vi "Pulse RFSG.vi"(0 "Test Configuration":T5, 5 "RFmx Settings":T1={"Center Frequency (Hz)"=10000000000.0, "Measurement Bandwidth (Hz)"=80000000.0, "Reference Level (dBm)"=10.0, "RFmx De-embedding"={"RFmx Name"="5842_0", "RFmx Port"="", "Attenuation"={"Mode"=enum."Constant Attenuation", "Constant Attenuation"={"RFmx External Attenuation (dB)"=1.2}, "s2p File"={"RFmx S-Parameters Orientation"=24000, "RFmx Attenuation s2p Path Name"="", "RFmx Attenuation s2p File"=path ""}}}, "Acquisition Length (s)"=0.0} {"RFmx De-embedding"."Attenuation"."s2p File"."RFmx S-Parameters Orientation" items=["Port1 Towards DUT"=24000, "Port2 Towards DUT"=24001]; "RFmx De-embedding"."Attenuation"."Constant Attenuation"."RFmx External Attenuation (dB)" format="%.2f"; "Reference Level (dBm)" format="%.2f"; "Measurement Bandwidth (Hz)" format="%.3p"; "Center Frequency (Hz)" format="%.6p"}, 7 "RFSG settings":T3={"RFSG De-embedding"={"RFSG Name"="5842_0", "RFSG Port"="", "Attenuation"={"Mode"=enum."Constant Attenuation", "Contant Attenuation"={"RFSG External Attenuation (dB)"=2.0}, "s2p File"={"RFSG S-parameters Orientation"=24000, "RFSG Attenuation s2p Path Name"="", "RFSG s2p File Path"=path ""}}}, "Generation IQ Rate (S/s)"=0.0} {"RFSG De-embedding"."Attenuation"."s2p File"."RFSG S-parameters Orientation" items=["Port1 Towards DUT"=24000, "Port2 Towards DUT"=24001]; "RFSG De-embedding"."Attenuation"."Contant Attenuation"."RFSG External Attenuation (dB)" format="%.2f"}, 11 "error in":errorcluster) -> (4 "RFSG session":refnum<k15>, 15 "error out":errorcluster)   [LabVIEW 2023]
uses:
  Controls/Test Config - Pulse.ctl
  Controls/RFSG Config - Pulse.ctl
  FPT Shared VIs/De-embedding/RFsg Config.ctl
  Controls/RFmx Config - Pulse.ctl
  FPT Shared VIs/De-embedding/RFmx Config.ctl
  <instrlib>/niRFSG/niRFSG.llb/niRFSG Write Arb Waveform (Complex DBL).vi
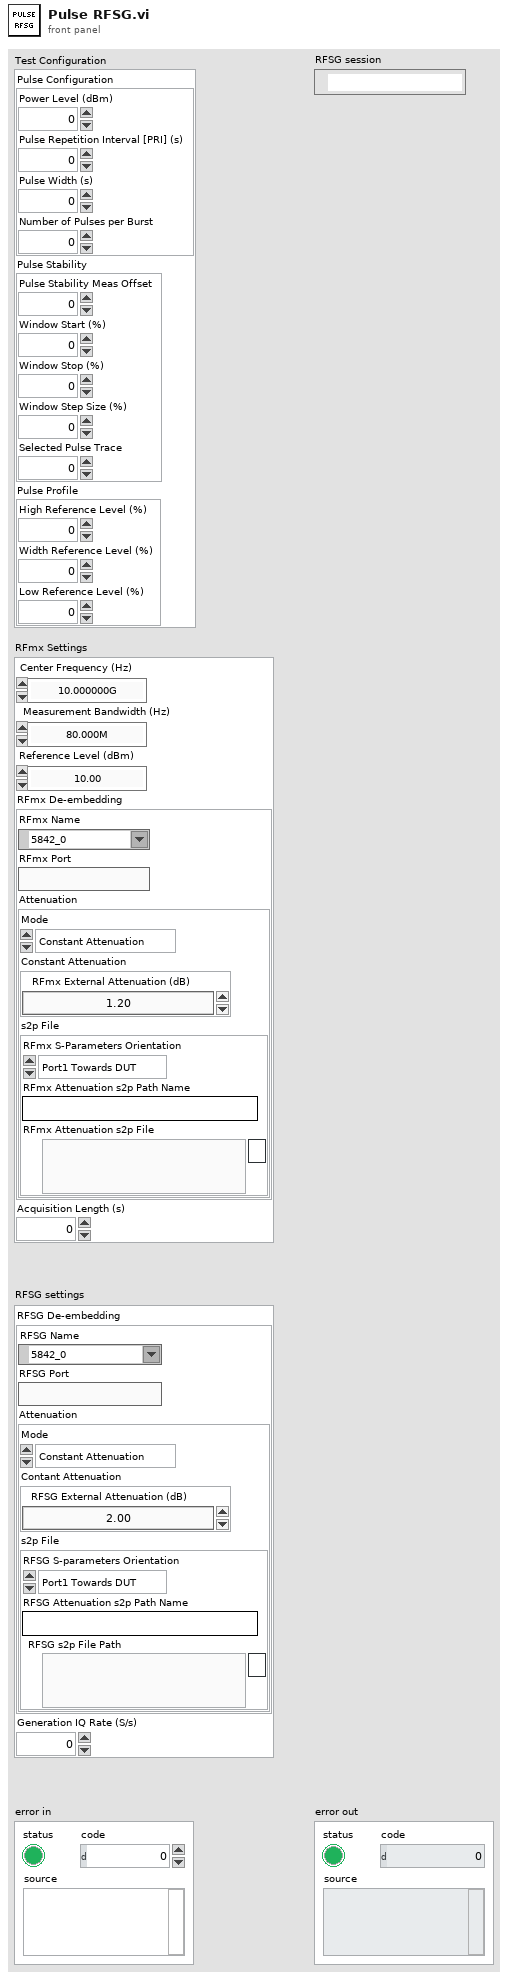
[diagram p1: front panel]
types:
  T1 = typedef "RFmx Config - Pulse.ctl" = cluster{"Center Frequency (Hz)":dbl, "Measurement Bandwidth (Hz)":dbl, "Reference Level (dBm)":dbl, "RFmx De-embedding":T2, "Acquisition Length (s)":dbl}
  T2 = typedef "RFmx Config.ctl" = cluster{"RFmx Name":refnum<k15>, "RFmx Port":string, "Attenuation":cluster{"Mode":enum32{"<None>", "Constant Attenuation", "s2p File"}, "Constant Attenuation":cluster{"RFmx External Attenuation (dB)":dbl}, "s2p File":cluster{"RFmx S-Parameters Orientation":i32, "RFmx Attenuation s2p Path Name":string, "RFmx Attenuation s2p File":path}}}
  T3 = typedef "RFSG Config - Pulse.ctl" = cluster{"RFSG De-embedding":T4, "Generation IQ Rate (S/s)":dbl}
  T4 = typedef "RFsg Config.ctl" = cluster{"RFSG Name":refnum<k15>, "RFSG Port":string, "Attenuation":cluster{"Mode":enum32{"<None>", "Constant Attenuation", "s2p File"}, "Contant Attenuation":cluster{"RFSG External Attenuation (dB)":dbl}, "s2p File":cluster{"RFSG S-parameters Orientation":i32, "RFSG Attenuation s2p Path Name":string, "RFSG s2p File Path":path}}}
  T5 = typedef "Test Config - Pulse.ctl" = cluster{"Pulse Configuration":cluster{"Power Level (dBm)":dbl, "Pulse Repetition Interval [PRI] (s)":dbl, "Pulse Width (s)":dbl, "Number of Pulses per Burst":u32}, "Pulse Stability":cluster{"Pulse Stability Meas Offset":i32, "Window Start (%)":dbl, "Window Stop (%)":dbl, "Window Step Size (%)":dbl, "Selected Pulse Trace":i32}, "Pulse Profile":cluster{"High Reference Level (%)":dbl, "Width Reference Level (%)":dbl, "Low Reference Level (%)":dbl}}
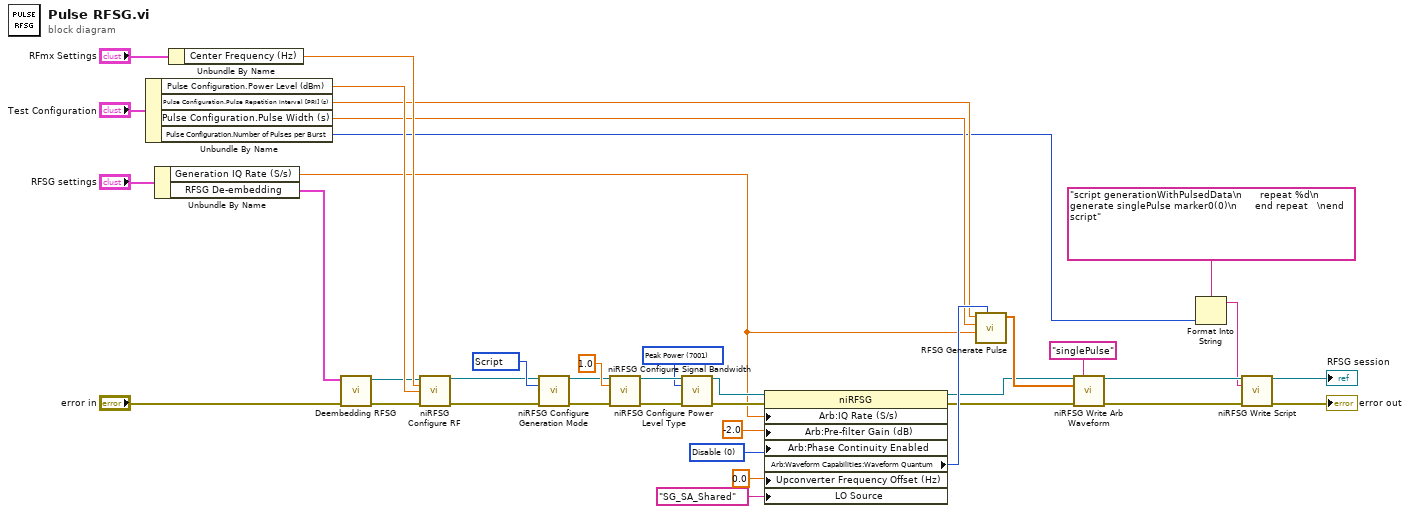
[diagram p0: block diagram]
diagram:
  w24 = 7001 items=["Average Power"=7000, "Peak Power"=7001] ("power level type")
  w33 = 0 items=["Auto"=-1, "Disable"=0, "Enable"=1] ("Arb Waveform:Phase Continuity Enabled")
  w36 = 1002 items=["CW"=1000, "Arb Waveform"=1001, "Script"=1002] ("generation mode")
  n1 = Unbundle By Name("Test Configuration") -> ("Pulse Configuration.Power Level (dBm)"=w15:dbl, "Pulse Configuration.Pulse Repetition Interval [PRI] (s)"=w14:dbl, "Pulse Configuration.Pulse Width (s)"=w13:dbl, "Pulse Configuration.Number of Pulses per Burst"=w11:u32)
  n2 = Unbundle By Name("RFSG settings") -> ("Generation IQ Rate (S/s)"=w12:dbl, "RFSG De-embedding"=w5:T4)
  n3 = Unbundle By Name("RFmx Settings") -> ("Center Frequency (Hz)"=w17:dbl)
  n4 = call "Deembedding RFSG.vi"("error in"="error in", "RFSG Settings"=w5) -> ("error out"=w8:errorcluster, "IVI Refnum out"=w6:refnum<k15>)  [unwired: 8 in]
  n5 = call <instrlib>:"niRFSG Configure RF.vi"("instrument handle"=w6, "frequency (Hz)"=w17, "power level (dBm)"=w15, "error in"=w8) -> ("instrument handle out"=w20:refnum<k15>, "error out"=w21:errorcluster)  [unwired: 10 in]
  n6 = call <instrlib>:"niRFSG Configure Generation Mode.vi"("instrument handle"=w20, "generation mode"=w36, "error in"=w21) -> ("instrument handle out"=w30:refnum<k15>, "error out"=w29:errorcluster)  [unwired: 11 in]
  n7 = call <instrlib>:"niRFSG Configure Signal Bandwidth.vi"("instrument handle"=w30, "signal bandwidth (Hz)"=1.0 ("x"), "error in"=w29) -> ("instrument handle out"=w28:refnum<k15>, "error out"=w26:errorcluster)  [unwired: 11 in]
  n8 = call <instrlib>:"niRFSG Configure Power Level Type.vi"("instrument handle"=w28, "power level type"=w24, "error in"=w26) -> ("instrument handle out"=w27:refnum<k15>, "error out"=w25:errorcluster)  [unwired: 11 in]
  n9 = property class="niRFSG"(reference=w27, error in=w25, "Arb:IQ Rate (S/s)"=w12, "Arb:Pre-filter Gain (dB)"=-2.0 ("RF:Advanced:AWG:DUC Pre-filter Gain (dB)"), "Arb:Phase Continuity Enabled"=w33, "Upconverter Frequency Offset (Hz)"=0.0 ("Device Specific:Vector Signal Transceiver:Upconverter:Frequency Offset (Hz)"), "LO Source"="SG_SA_Shared" ("Device Specific:Vector Signal Transceiver:Signal Path:LO Source")) -> (reference out=w4:refnum<k15>, error out=w3:errorcluster, "Arb:Waveform Capabilities:Waveform Quantum"=w22:i32)
  n10 = call "RFSG Generate Pulse.vi"("quantum"=w22, "IQ Rate (S/s)"=w12, "Pulse Width (s)"=w13, "Pulse Repetition Interval [PRI] (s)"=w14) -> ("IQ - Single Pulse"=w23:cdb[])  [unwired: 7 in]
  n11 = call-poly <instrlib>:"niRFSG Write Arb Waveform.vi"("instrument handle"=w4, "name"="singlePulse", "waveform data"=w23, "error in"=w3) -> ("instrument handle out"=w38:refnum<k15>, "error out"=w37:errorcluster)  [unwired: 10 in]
  n12 = Format Into String(format string="script generationWithPulsedData\n      repeat %d\n         generate singlePulse marker0(0)\n      end repeat   \nend script" ("script"), w11) -> (resulting string=w34:string)  [unwired: 2 in, 1 out]
  n13 = call <instrlib>:"niRFSG Write Script.vi"("instrument handle"=w38, "script"=w34, "error in"=w37) -> ("instrument handle out"=→"RFSG session":refnum<k15>, "error out"=→"error out":errorcluster)  [unwired: 11 in]
